vi "LockBit_HT.vi"(8 "error in (no error)":errorcluster) -> (0 "error out":errorcluster, 3 "HT Lock Result":bool)   [LabVIEW 2011]
doc: "This VI reads the lock bit state for the HT PLL.\n\nOutputs:\n1. HT Lock Result: The lock bit result for the HT PLL (1 locked or 0 unlocked)."
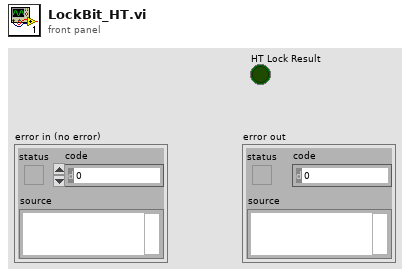
[diagram p1: front panel]
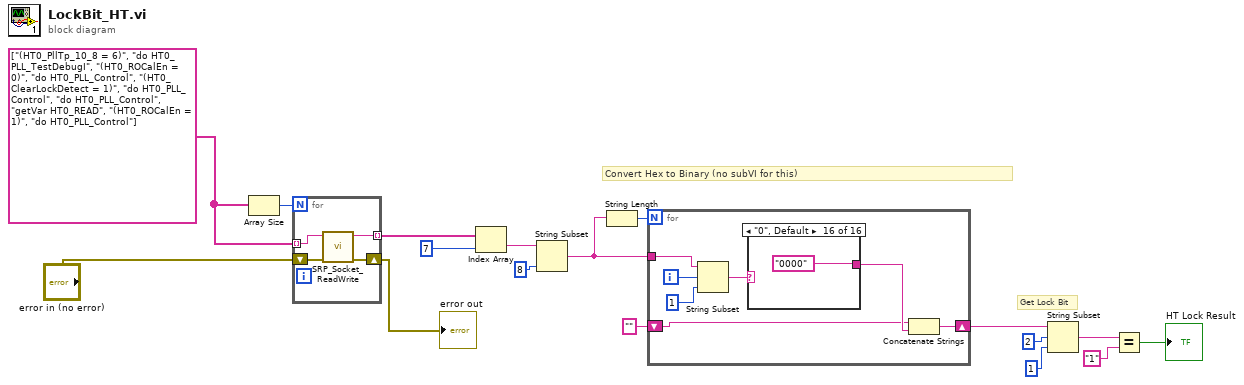
[diagram p0: block diagram]
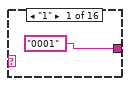
[diagram p2: hidden frame]
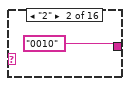
[diagram p3: hidden frame]
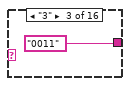
[diagram p4: hidden frame]
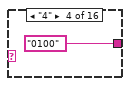
[diagram p5: hidden frame]
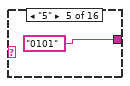
[diagram p6: hidden frame]
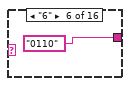
[diagram p7: hidden frame]
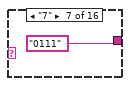
[diagram p8: hidden frame]
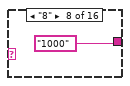
[diagram p9: hidden frame]
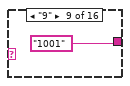
[diagram p10: hidden frame]
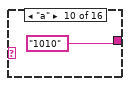
[diagram p11: hidden frame]
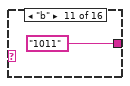
[diagram p12: hidden frame]
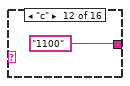
[diagram p13: hidden frame]
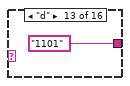
[diagram p14: hidden frame]
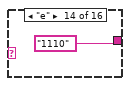
[diagram p15: hidden frame]
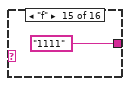
[diagram p16: hidden frame]
diagram:
  w16 = string[] ["(HT0_PllTp_10_8 = 6)", "do HT0_PLL_TestDebugI", "(HT0_ROCalEn =  0)", "do HT0_PLL_Control", "(HT0_ClearLockDetect = 1)", "do HT0_PLL_Control", "do HT0_PLL_Control", "getVar HT0_READ", "(HT0_ROCalEn =  1)", "do HT0_PLL_Control"]
  # "Get Lock Bit"
  # "Convert Hex to Binary (no subVI for this)"
  n1 = Array Size(array=w16) -> (size(s)=w17:i32)
  n2 = for {
    N: w17 -> [_]
    shift-right: [w20] -> w13
    shift-left: "error in (no error)" -> [w21]
    tunnel: w16 -> [w19] mode=indexing
    tunnel: [w18] -> w15 mode=indexing
    n3 = call "SRP_Socket_ReadWrite.vi"("error in (no error)"=w21, "Data In"=w19) -> ("error out"=w20:errorcluster, "Data Out"=w18:string)  [unwired: 7 in]
  }
  "error out" <- w13
  n4 = Index Array(array=w15, index=7) -> (element=w8:string)
  n5 = String Subset(string=w8, length (rest)=8 ("length (rest)")) -> (substring=w7:string)  [unwired: 1 in]
  n6 = String Length(string=w7) -> (length=w11:i32)
  n7 = for {
    N: w11 -> [_]
    tunnel: w7 -> [w27]
    shift-right: [w24] -> w4
    shift-left: "" -> [w22]
    i -> [w25]
    n8 = String Subset(string=w27, offset (0)=w25, length (rest)=1 ("length (rest)")) -> (substring=w28:string)
    n9 = case shown="\"0\", Default" w28 {
      tunnel: ["0001" "0010" "0011" "0100" "0101" "0110" "0111" "1000" "1001" "1010" "1011" "1100" "1101" "1110" "1111" "0000"] -> w23
      frame "1" {
      }
      frame "2" {
      }
      frame "3" {
      }
      frame "4" {
      }
      frame "5" {
      }
      frame "6" {
      }
      frame "7" {
      }
      frame "8" {
      }
      frame "9" {
      }
      frame "a" {
      }
      frame "b" {
      }
      frame "c" {
      }
      frame "d" {
      }
      frame "e" {
      }
      frame "f" {
      }
      frame "0", Default {
      }
    }
    n10 = Concatenate Strings(w22, w23) -> (w24:string)
  }
  n11 = String Subset(string=w4, offset (0)=2, length (rest)=1 ("length (rest)")) -> (substring=w1:string)
  n12 = Equal?(x=w1, y="1") -> (x = y?=→"HT Lock Result":bool)
